vi "5-v1v2.vi"(3 "this":i32, 4 "button":i32, 5 "shift in":bool) -> (0 "next state":i32, 1 "shift out":bool)   [LabVIEW 2017]
panel:
  out "setting out":T1
  in  "setting in":T1={"Auto1"=TRUE, "Auto2"=TRUE, "Rel1"=TRUE, "Rel2"=TRUE, "Filt1"=TRUE, "Filt2"=TRUE, "Rate"=enum."Slow", "Range1"=enum."10mV", "Range2"=enum."100mV", "Filt3"=TRUE, "Filt4"=TRUE, "Rel temp 1"=TRUE, "Analog1"=FALSE, "Analog2"=FALSE, "Analog temp 1"=FALSE, "Digital1"=TRUE, "Digital2"=TRUE, "Digital temp 1 "=TRUE, "Window1"=enum."0,01%", "Window2"=enum."0,01%", "Window temp 1"=enum."0,01%", "RDGS1"="010", "RDGS2"="010", "RDGS temp 1"="010", "Type_type1"=TRUE, "Type_type2"=TRUE, "Type_type temp 1"=TRUE, "LSync"=FALSE, "Unit"=enum."C", "Sens"=TRUE, "Type tcoupl"=enum."J", "Junc"=TRUE, "prevState"=0, "Rel temp 2"=TRUE, "Analog temp 2"=FALSE, "Digital temp 2"=TRUE, "Type_type temp 2"=TRUE, "RDGS temp 2"="010", "Window temp 2"=enum."0,01%", "addres"="0"}
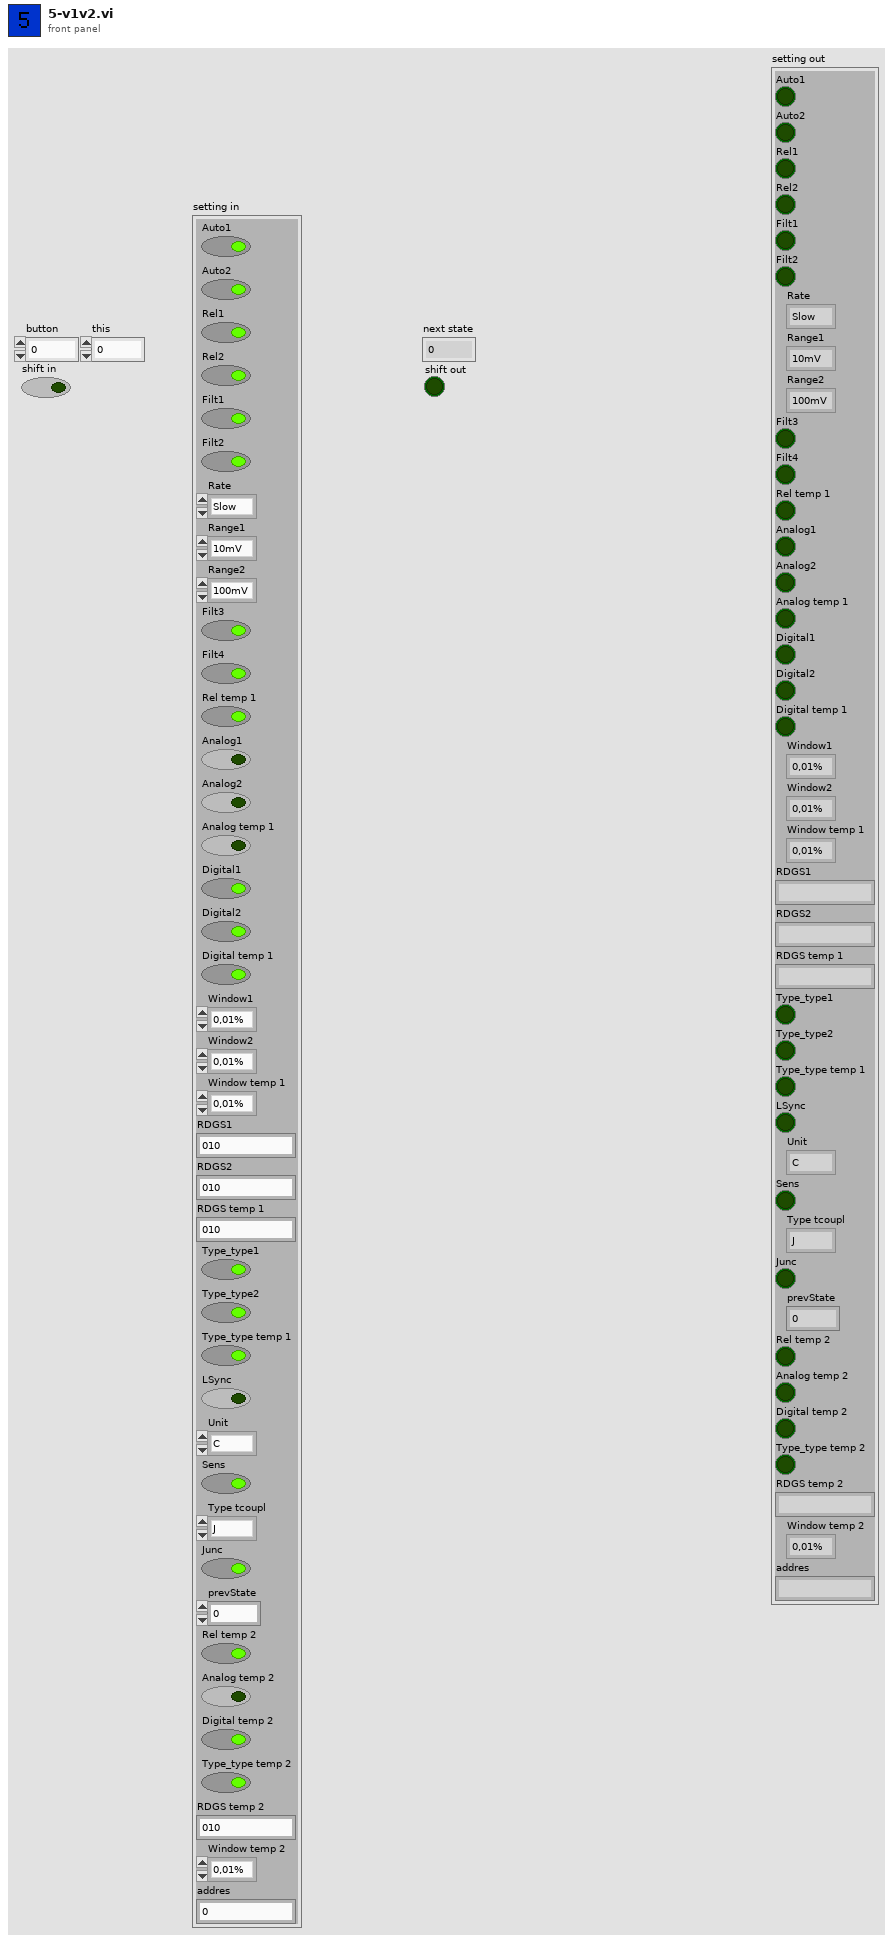
[diagram p1: front panel]
types:
  T1 = cluster{"Auto1":bool, "Auto2":bool, "Rel1":bool, "Rel2":bool, "Filt1":bool, "Filt2":bool, "Rate":enum16{"Slow", "Med", "Fast"}, "Range1":enum16{"10mV", "100mV", "1V", "10V", "100V"}, "Range2":enum16{"100mV", "1V", "10V"}, "Filt3":bool, "Filt4":bool, "Rel temp 1":bool, "Analog1":bool, "Analog2":bool, "Analog temp 1":bool, "Digital1":bool, "Digital2":bool, "Digital temp 1 ":bool, "Window1":enum16{"0,01%", "0,1%", "1%", "10%", "None"}, "Window2":enum16{"0,01%", "0,1%", "1%", "10%", "None"}, "Window temp 1":enum16{"0,01%", "0,1%", "1%", "10%", "None"}, "RDGS1":string, "RDGS2":string, "RDGS temp 1":string, "Type_type1":bool, "Type_type2":bool, "Type_type temp 1":bool, "LSync":bool, "Unit":enum16{"C", "K", "F"}, "Sens":bool, "Type tcoupl":enum16{"J", "K", "T", "E", "R", "S", "B", "N"}, "Junc":bool, "prevState":i32, "Rel temp 2":bool, "Analog temp 2":bool, "Digital temp 2":bool, "Type_type temp 2":bool, "RDGS temp 2":string, "Window temp 2":enum16{"0,01%", "0,1%", "1%", "10%", "None"}, "addres":string}
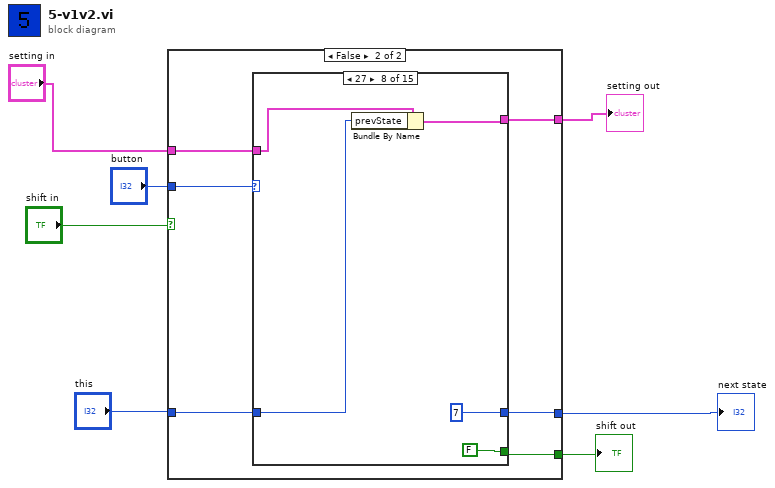
[diagram p0: block diagram]
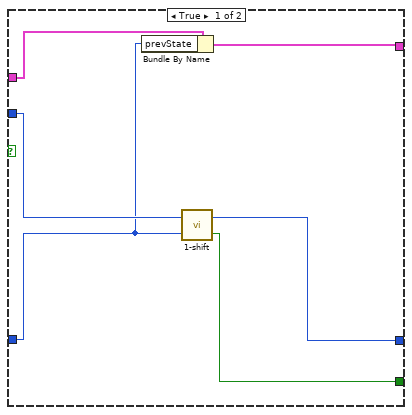
[diagram p2: hidden frame]
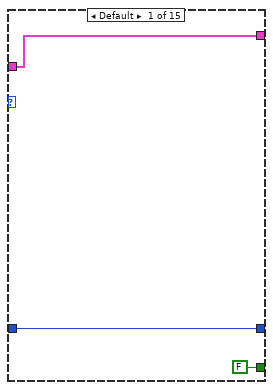
[diagram p3: hidden frame]
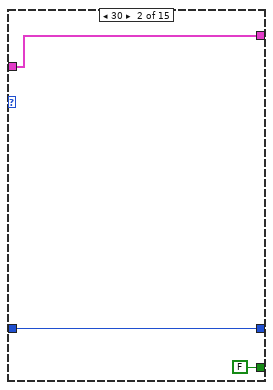
[diagram p4: hidden frame]
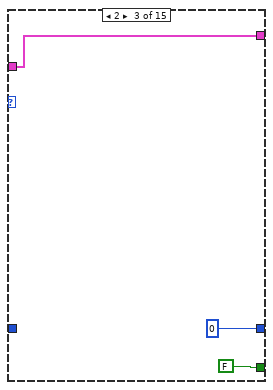
[diagram p5: hidden frame]
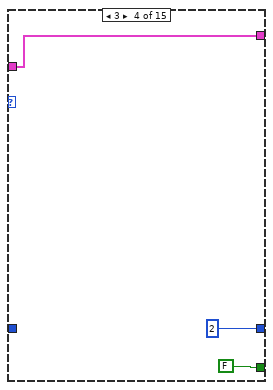
[diagram p6: hidden frame]
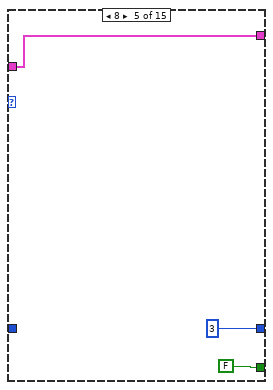
[diagram p7: hidden frame]
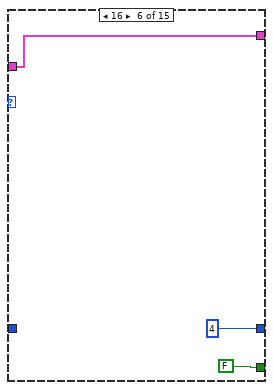
[diagram p8: hidden frame]
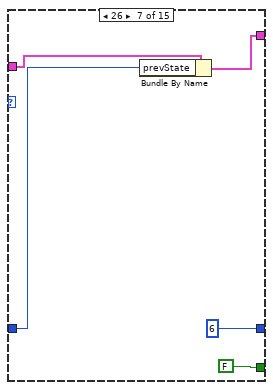
[diagram p9: hidden frame]
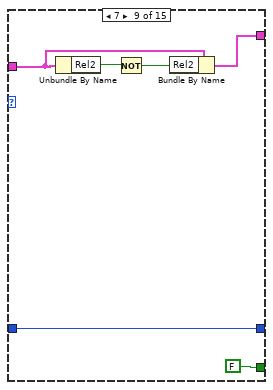
[diagram p10: hidden frame]
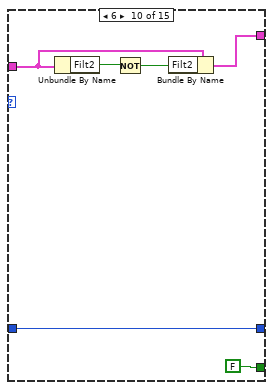
[diagram p11: hidden frame]
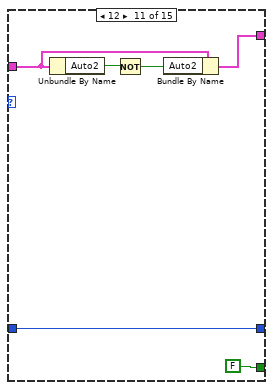
[diagram p12: hidden frame]
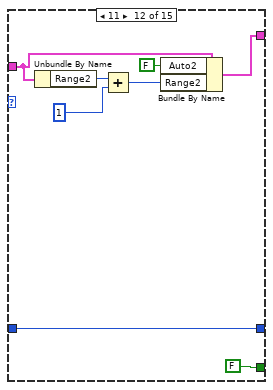
[diagram p13: hidden frame]
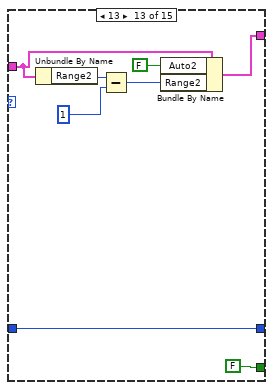
[diagram p14: hidden frame]
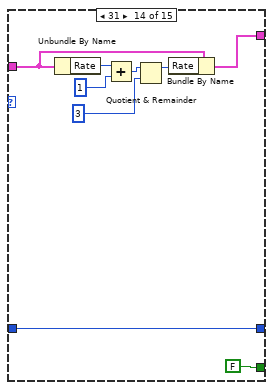
[diagram p15: hidden frame]
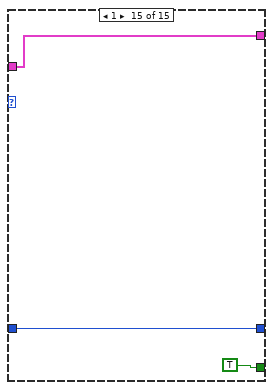
[diagram p16: hidden frame]
diagram:
  n1 = case shown="False" "shift in" {
    tunnel: "button" -> [w13 w19]
    tunnel: [w12 w18] -> w5
    tunnel: "this" -> [w8 w17]
    tunnel: [w11 w16] -> w3
    tunnel: [w9 w15] -> w1
    tunnel: "setting in" -> [w10 w14]
    frame True {
      n2 = Bundle By Name(cluster=w10, "prevState"=w8) -> (w9:T1)
      n3 = call "1-shift.vi"("this"=w8, "button"=w13) -> ("shift"=w11:bool, "next state"=w12:i32)
    }
    frame False {
      n4 = case shown="27" w19 {
        tunnel: [w22 w25 0 2 3 4 6 7 w52 w58 w64 w72 w80 w89 w93] -> w18
        tunnel: w17 -> [w22 w25 _ _ _ _ w38 w45 w52 w58 w64 w72 w80 w89 w93]
        tunnel: [FALSE ("shift") FALSE ("shift") FALSE ("shift") FALSE ("shift") FALSE ("shift") FALSE ("shift") FALSE ("shift") FALSE ("shift") FALSE ("shift") FALSE ("shift") FALSE ("shift") FALSE ("shift") FALSE ("shift") FALSE ("shift") TRUE ("shift")] -> w16
        tunnel: [w20 w23 w26 w29 w32 w35 w39 w43 w50 w56 w62 w71 w79 w88 w91] -> w15
        tunnel: w14 -> [w20 w23 w26 w29 w32 w35 w40 w44 w49 w55 w61 w67 w75 w83 w91]
        frame Default {
        }
        frame 30 {
        }
        frame 2 {
        }
        frame 3 {
        }
        frame 8 {
        }
        frame 16 {
        }
        frame 26 {
          n5 = Bundle By Name(cluster=w40, "prevState"=w38) -> (w39:T1)
        }
        frame 27 {
          n6 = Bundle By Name(cluster=w44, "prevState"=w45) -> (w43:T1)
        }
        frame 7 {
          n7 = Unbundle By Name(w49) -> ("Rel2"=w48:bool)
          n8 = Not(x=w48) -> (.not. x?=w51:bool)
          n9 = Bundle By Name(cluster=w49, "Rel2"=w51) -> (w50:T1)
        }
        frame 6 {
          n10 = Unbundle By Name(w55) -> ("Filt2"=w54:bool)
          n11 = Not(x=w54) -> (.not. x?=w57:bool)
          n12 = Bundle By Name(cluster=w55, "Filt2"=w57) -> (w56:T1)
        }
        frame 12 {
          n13 = Unbundle By Name(w61) -> ("Auto2"=w60:bool)
          n14 = Not(x=w60) -> (.not. x?=w63:bool)
          n15 = Bundle By Name(cluster=w61, "Auto2"=w63) -> (w62:T1)
        }
        frame 11 {
          n16 = Unbundle By Name(w67) -> ("Range2"=w66:enum16{"100mV", "1V", "10V"})
          n17 = Add(x=w66, y=1) -> (x+y=w69:i32)
          n18 = Bundle By Name(cluster=w67, "Auto2"=FALSE ("Auto1"), "Range2"=w69) -> (w71:T1)
        }
        frame 13 {
          n19 = Unbundle By Name(w75) -> ("Range2"=w74:enum16{"100mV", "1V", "10V"})
          n20 = Subtract(x=w74, y=1) -> (x-y=w77:i32)
          n21 = Bundle By Name(cluster=w75, "Auto2"=FALSE ("Auto1"), "Range2"=w77) -> (w79:T1)
        }
        frame 31 {
          n22 = Unbundle By Name(w83) -> ("Rate"=w82:enum16{"Slow", "Med", "Fast"})
          n23 = Add(x=w82, y=1) -> (x+y=w86:i32)
          n24 = Quotient & Remainder(x=w86, y=3) -> (x-y*floor(x/y)=w85:i32)  [unwired: 1 out]
          n25 = Bundle By Name(cluster=w83, "Rate"=w85) -> (w88:T1)
        }
        frame 1 {
        }
      }
    }
  }
  "next state" <- w5
  "shift out" <- w3
  "setting out" <- w1
